vi "Newton Raphson Zero Finder.vi"   [LabVIEW 2024, in "NI_Gmath.lvlib"]
doc: "<p>Determines a zero of a 1D function close to two points with the help of the derivative of this 1D function. The two values form a search limit for the unknown zero of the 1D function. You must <a href=\"nihelplauncher://docs/csh?context=lvcore_lvhowto_selectingdefaultinstpolyvi\">manually select the polymorphic instance</a> to use.</p>"
uses:
  NI_Gmath.lvlib
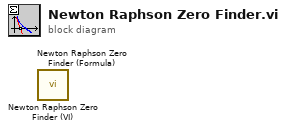
[diagram p0: block diagram]
diagram:
  n1 = call "Newton Raphson Zero Finder (VI).vi"() -> ()  [unwired: 8 in, 4 out]
  n2 = call "Newton Raphson Zero Finder (Formula).vi"() -> ()  [unwired: 8 in, 4 out]
